vi "globalSetUp.vi"(8 "error in":errorcluster, 11 "Single Core Simple Loopback in":refnum<class "Single Core Simple Loopback.lvclass">) -> (0 "error out":errorcluster, 3 "Single Core Simple Loopback out":refnum<class "Single Core Simple Loopback.lvclass">)   [LabVIEW 2020, in "Single Core Simple Loopback.lvclass"]
uses:
  Single Core Simple Loopback.lvclass
  niveristand-custom-device-testing-tools/VeriStandTestUtilities/VeriStandTestUtilities.lvlib
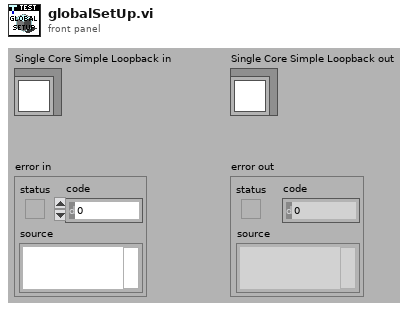
[diagram p1: front panel]
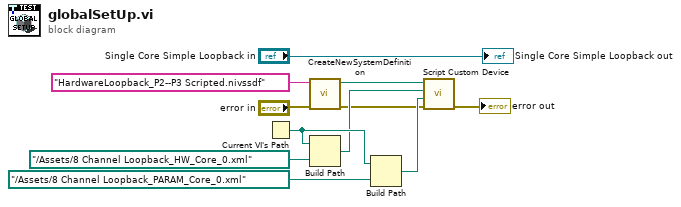
[diagram p0: block diagram]
diagram:
  n1 = Current VI's Path() -> (path=w11:path)
  n2 = call "CreateNewSystemDefinition.vi"("error in"="error in", "System Definition Name"="HardwareLoopback_P2--P3 Scripted.nivssdf" ("Channel")) -> ("error out"=w2:errorcluster, "System Definition Path"=w1:path)  [unwired: 8 in]
  n3 = Build Path(base path=w11, name or relative path=path "../Assets/8 Channel Loopback_HW_Core_0.xml" ("Hardware File Path")) -> (appended path=w10:path)
  n4 = Build Path(base path=w11, name or relative path=path "../Assets/8 Channel Loopback_PARAM_Core_0.xml" ("Hardware File Path")) -> (appended path=w9:path)
  n5 = call "Script Custom Device.vi"("error in"=w2, "Parameter File Path"=w9, "Hardware File Path"=w10, "System Definition File Path In"=w1) -> ("error out"=→"error out":errorcluster)  [unwired: 6 in, 1 out]
  "Single Core Simple Loopback out" <- "Single Core Simple Loopback in"
